vi "Log Data to File.vi"(7 "Data Cluster":T1, 8 "error in":errorcluster, 10 "Waveform":waveform(dbl), 11 "TDMS File Reference":refnum<k34>) -> (0 "error out":errorcluster)   [LabVIEW 2025, in "Logger.lvlib"]
doc: "This VI uses the TDMS Write function to write data to a TDMS file.\n_____\nBased on DQMH Dev Tools: Project Template 7.1.0.1503."
uses:
  Logger.lvlib
  Module Data--cluster.ctl
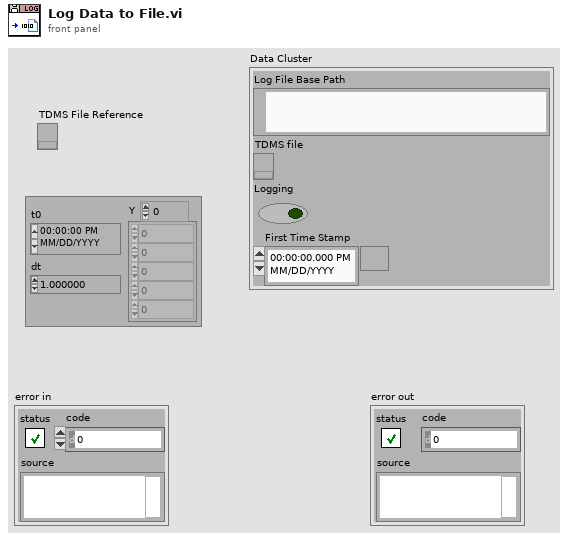
[diagram p1: front panel]
types:
  T1 = typedef "Logger.lvlib/Module Data--cluster.ctl" = cluster{"Log File Base Path":path, "TDMS file":refnum<k34>, "Logging":bool, "First Time Stamp":timestamp}
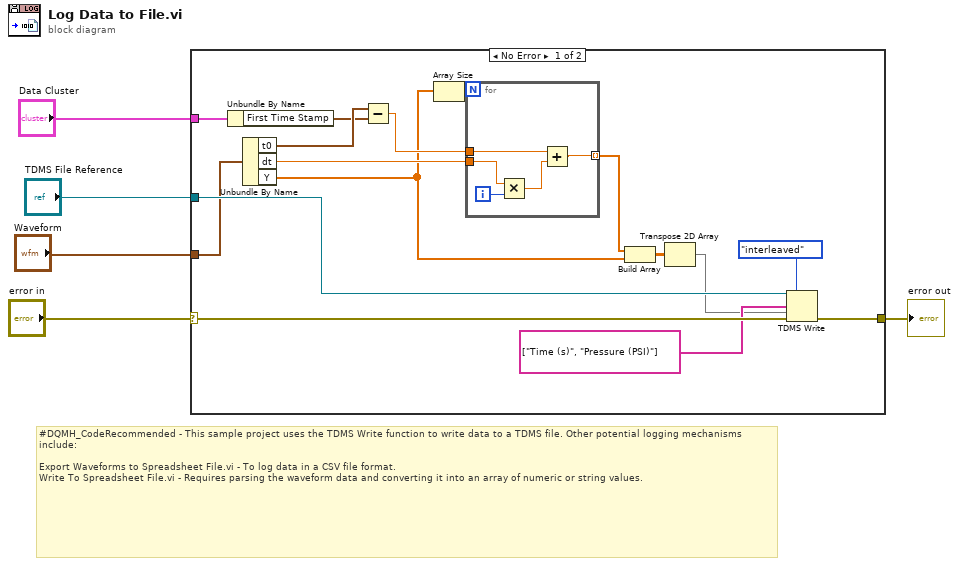
[diagram p0: block diagram]
diagram:
  # "#DQMH_CodeRecommended - This sample project uses the TDMS Write function to write data to a TDMS file. Other potential logging mechanisms include:\n\nExport Waveforms to Spreadsheet File.vi - To log data in a CSV file format.\nWrite To Spreadsheet File.vi - Requires parsing the waveform data and converting it into an array of numeric or string values."
  n1 = case shown="No Error" "error in" {
    selector: "error in" -> [w20 w27]
    tunnel: "Waveform" -> [w17 _]
    tunnel: [w21 w27] -> w5
    tunnel: "TDMS File Reference" -> [w19 _]
    tunnel: "Data Cluster" -> [w18 _]
    frame No Error {
      n2 = Unbundle By Name(w18) -> ("First Time Stamp"=w15:timestamp)
      n3 = Unbundle By Name(w17) -> ("t0"=w16:timestamp, "dt"=w13:dbl, "Y"=w10:dbl[])
      n4 = Subtract(x=w16, y=w15) -> (x-y=w12:dbl)
      n5 = Array Size(array=w10) -> (size(s)=w14:i32)
      n6 = for {
        N: w14 -> [_]
        tunnel: w13 -> [w23]
        tunnel: w12 -> [w26]
        tunnel: [w25] -> w11 mode=indexing
        i -> [w24]
        n7 = Multiply(x=w23, y=w24) -> (x*y=w22:dbl)
        n8 = Add(x=w26, y=w22) -> (x+y=w25:dbl)
      }
      n9 = Build Array(w11, w10) -> (w9:dbl[][])
      n10 = Transpose 2D Array(2D array=w9) -> (transposed array=w6:dbl[][])
      n11 = TDMS Write(0:w19, 1:enum16{"decimated", "interleaved"}."interleaved" ("data layout (0:decimated)"), 7:string[] ["Time (s)", "Pressure (PSI)"] ("channel name(s) in (Untitled)"), 9:w6, 11:w20) -> (15:w21:errorcluster)  [unwired: 1 in, 3 out]
    }
    frame Error {
    }
  }
  "error out" <- w5
